vi "Configure DC Volts.vi"(5 "NPLC (1)":dbl=1.0 min=0.001 max=10.0, 7 "Range (Auto)":T1(ring), 8 "error in":errorcluster, 9 "Digits (7.5)":enum16{"3.5", "4.5", "5.5", "6.5", "7.5"}(ring)=enum."7.5", 10 "Channel (Channel 1)":enum16{"Channel 1", "Channel 2"}(ring), 11 "VISA resource name":refnum<visa-resource-name>) -> (0 "error out":errorcluster, 3 "VISA resource name out":refnum<visa-resource-name>)   [LabVIEW 2016, in "Keithley 2182A.lvlib"]
uses:
  <instrlib>/Keithley 2182A/Keithley 2182A.lvlib
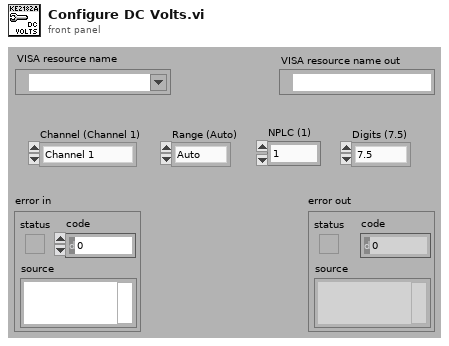
[diagram p1: front panel]
types:
  T1 = enum16{"Auto", "10 mV", "100 mV", "1 V", "10 V", "100 V"}
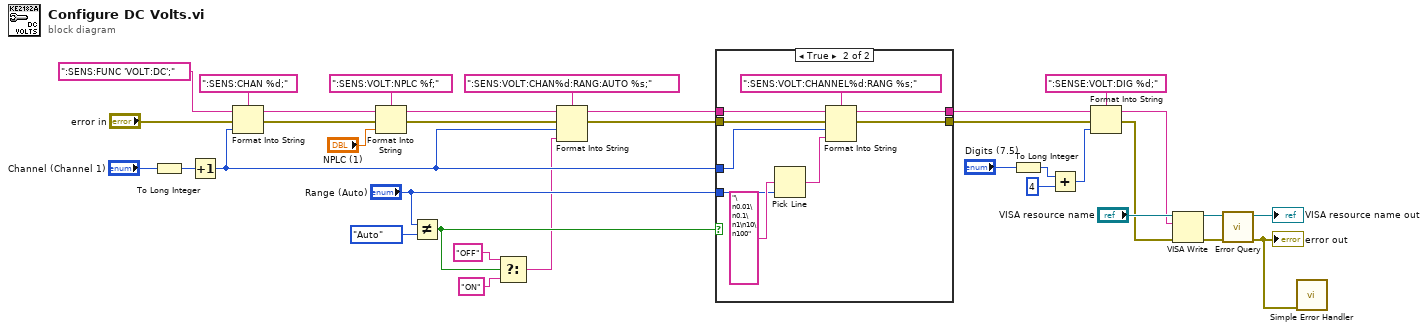
[diagram p0: block diagram]
diagram:
  n1 = To Long Integer(number="Channel (Channel 1)") -> (32bit integer=w17:i32)
  n2 = Increment(x=w17) -> (x+1=w15:i32)
  n3 = Format Into String(format string=":SENS:CHAN %d;", initial string=":SENS:FUNC 'VOLT:DC';" ("format string"), error in="error in", w15) -> (resulting string=w28:string, error out=w29:errorcluster)
  n4 = Format Into String(format string=":SENS:VOLT:NPLC %f;", initial string=w28, error in=w29, "NPLC (1)") -> (resulting string=w22:string, error out=w21:errorcluster)
  n5 = Not Equal?(x="Range (Auto)", y=T1."Auto") -> (x != y?=w11:bool)
  n6 = Select(t="OFF", s=w11, f="ON") -> (s? t:f=w10:string)
  n7 = Format Into String(format string=":SENS:VOLT:CHAN%d:RANG:AUTO %s;", initial string=w22, error in=w21, w15, w10) -> (resulting string=w23:string, error out=w20:errorcluster)
  n8 = case shown="True" w11 {
    tunnel: [w37 w45] -> w24
    tunnel: w23 -> [w37 w44]
    tunnel: w20 -> [w36 w43]
    tunnel: [w36 w42] -> w19
    tunnel: w15 -> [_ w39]
    tunnel: "Range (Auto)" -> [_ w38]
    frame False {
    }
    frame True {
      n9 = Pick Line(multi-line string="\n0.01\n0.1\n1\n10\n100", line index=w38) -> (output string=w40:string)  [unwired: 1 out]
      n10 = Format Into String(format string=":SENS:VOLT:CHANNEL%d:RANG %s;", initial string=w44, error in=w43, w39, w40) -> (resulting string=w45:string, error out=w42:errorcluster)
    }
  }
  n11 = To Long Integer(number="Digits (7.5)") -> (32bit integer=w9:i32)
  n12 = Add(x=w9, y=4) -> (x+y=w6:i32)
  n13 = Format Into String(format string=":SENSE:VOLT:DIG %d;", initial string=w24, error in=w19, w6) -> (resulting string=w1:string, error out=w4:errorcluster)
  n14 = VISA Write(VISA resource name="VISA resource name", write buffer=w1, error in (no error)=w4) -> (VISA resource name out=w34:refnum<visa-resource-name>, error out=w35:errorcluster)  [unwired: 1 out]
  n15 = call <instrlib>:"Error Query.vi"("error in (no error)"=w35, "VISA resource name"=w34) -> ("error out"=w3:errorcluster, "VISA resource name out"=→"VISA resource name out":refnum<visa-resource-name>)  [unwired: 8 out]
  "error out" <- w3
  n16 = call <vilib>:"Simple Error Handler.vi"("error in (no error)"=w3) -> ()  [unwired: 1 in, 8 out]
